vi "Configure Multiple Tone Characteristics.vi"(6 "State (1: On)":u16(ring)=1 items=["Off", "On"], 7 "Power (0 dB)":dbl, 8 "error in (no error)":errorcluster, 9 "Phase (0 deg)":dbl, 10 "Row No. (1)":i32=1, 11 "VISA resource name":refnum<visa-resource-name>) -> (0 "error out":errorcluster, 3 "VISA resource name out":refnum<visa-resource-name>)   [LabVIEW 2011, in "Agilent PSG MXG Series.lvlib"]
doc: "Modifies the specific tone (row) of the multitone waveform.\n\n<B>Notes:</B>\n(1) This VI is valid only in E8267C, E8267D, N5182A.\n\n(2) For E8267C, this VI is valid only when the instrument installs <B>Option 002</B> (Internal baseband generator) or <B>Option 602</B> (Digital bus baseband generator).\n\n(3) For E8267D, this VI is valid only when the instrument installs <B>Option 601</B> or <B>Option 602</B> (Internal baseband generator).\n\n(4) For N5182A, this VI is valid only when the instrument installs <B>Option 651</B> or <B>Option 652</B> or <B>Option 654</B> (Internal baseband generator), and <B>Option 430</B> (Multitone and two-tone)."
uses:
  Agilent PSG MXG Series.lvlib
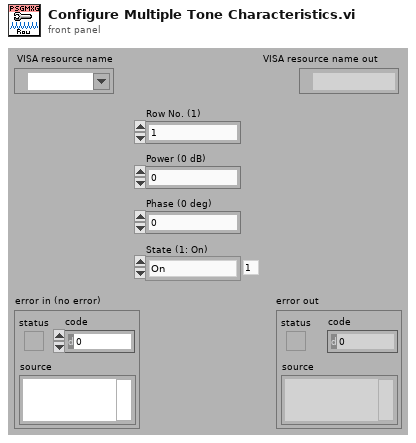
[diagram p1: front panel]
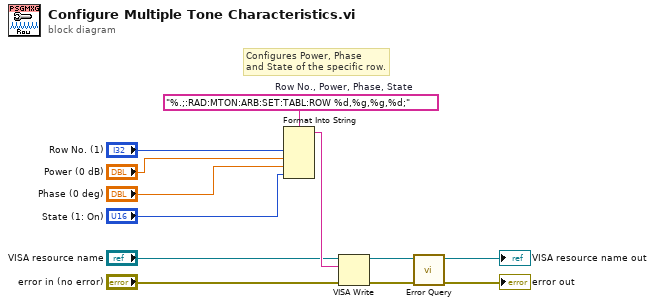
[diagram p0: block diagram]
diagram:
  w12 = "%.;:RAD:MTON:ARB:SET:TABL:ROW %d,%g,%g,%d;"  # Row No., Power, Phase, State
  # "Configures Power, Phase\nand State of the specific row."
  n1 = Format Into String(format string=w12, "Row No. (1)", "Power (0 dB)", "Phase (0 deg)", "State (1: On)") -> (resulting string=w7:string)  [unwired: 2 in, 1 out]
  n2 = VISA Write(VISA resource name="VISA resource name", write buffer=w7, error in (no error)="error in (no error)") -> (VISA resource name out=w6:refnum<visa-resource-name>, error out=w5:errorcluster)  [unwired: 1 out]
  n3 = call "Error Query.vi"("error in (no error)"=w5, "VISA resource name"=w6) -> ("error out"=→"error out":errorcluster, "VISA resource name out"=→"VISA resource name out":refnum<visa-resource-name>)  [unwired: 6 in, 2 out]
